vi "Test Latch when pressed.vi"(11 "Error in":errorcluster) -> (15 "Error out":errorcluster)   [LabVIEW 2020, in "Mechanical Actions Tests.lvlib"]
doc: "This VI is used to test latch when pressed function"
uses:
  Mechanical Actions Tests.lvlib
  <vilib>/addons/_JKI Toolkits/Caraya/classes/Test Suite/Define Test Suite (JUnit Report).vi
  <vilib>/SLL Drona/APIs/Stimulus/ControlValue/SetValueAuto.vi
  <vilib>/SLL Drona/APIs/Assert/AssertControlValue/Equal.vi
  <vilib>/SLL Drona/APIs/Stimulus/VI/CloseVI.vi
  <vilib>/Utility/error.llb/Error Cluster From Error Code.vi
  <vilib>/ErrorRing/Error Ring.xnode
  <vilib>/addons/_JKI Toolkits/Caraya/classes/Test Suite/Test Suite.lvclass
  <vilib>/addons/_JKI Toolkits/Caraya/classes/Test/Test.lvclass
  <vilib>/SLL Drona/Drona.lvlib
  <vilib>/SLL Drona/APIs/Stimulus/ControlValue/ControlValue.lvlib
  <vilib>/SLL Drona/APIs/Assert/AssertControlValue/AssertControlValue.lvlib
  <vilib>/Wiresmith Technology/G CLI/CLI Class/CLI.lvclass
  <vilib>/SLL Drona/APIs/Stimulus/VI/VI.lvlib
panel:
  # "LATCH WHEN PRESSED TEST"
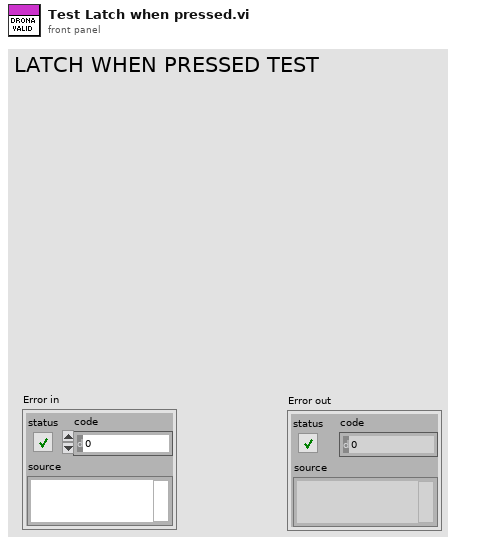
[diagram p1: front panel]
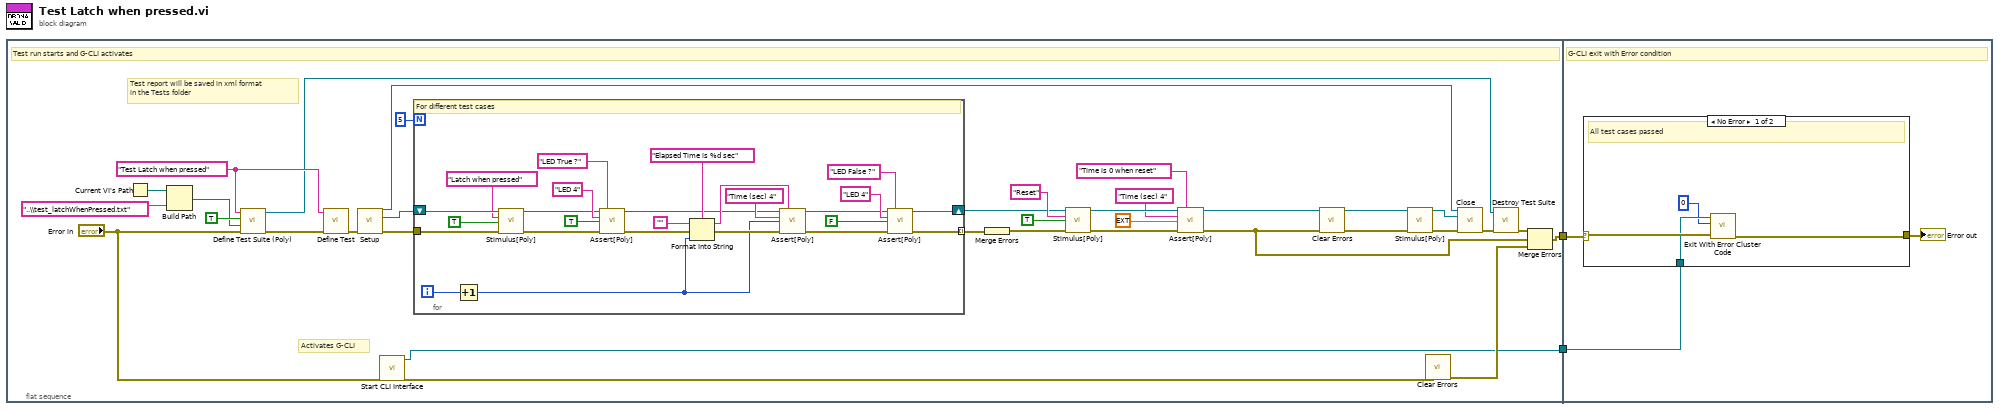
[diagram p0: block diagram]
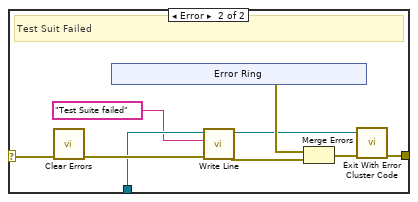
[diagram p2: hidden frame]
diagram:
  n1 = flat-sequence {
    tunnel: [w18] -> w2
    tunnel: [w5] -> w1
    tunnel: w2 -> [w64]
    tunnel: w1 -> [w62]
    frame #0 {
      w14 = "Test Latch when pressed" ("Label (VI Title)")
      # "Test report will be saved in xml format\nin the Tests folder"
      # "Activates G-CLI"
      # "Test run starts and G-CLI activates"
      n2 = Current VI's Path() -> (path=w12:path)
      n3 = Build Path(base path=w12, name or relative path="..\\test_latchWhenPressed.txt") -> (appended path=w10:path)
      n4 = call-poly <vilib>:"Define Test Suite (Poly).vi"("error in (no error)"="Error in", "Report Path"=w10, "Interactive"=TRUE, "Label (VI Title)"=w14) -> ("error out"=w16:errorcluster, "Test Suite"=w7:refnum<class "Test Suite.lvclass">)  [unwired: 5 in, 1 out]
      n5 = call <vilib>:"Define Test.vi"("error in (no error)"=w16, "Label (VI Title)"=w14) -> ("error out"=w36:errorcluster)  [unwired: 8 in, 1 out]
      n6 = call <vilib>:"Setup.vi"("error in"=w36) -> ("Application Ref"=w25:refnum<vi>, "VI Reference Out"=w35:refnum<vi>, "error out"=w23:errorcluster)  [unwired: 12 in]
      n7 = call <vilib>:"Start CLI Interface.vi"("error in (no error)"="Error in") -> ("error out"=w6:errorcluster, "CLI out"=w5:refnum<class "CLI.lvclass">)  [unwired: 7 in, 2 out]
      n8 = for {
        N: 5 -> [_]
        shift-right: [w37] -> w27
        shift-left: w35 -> [w60]
        tunnel: w23 -> [w61]
        tunnel: [w38] -> w26 mode=indexing
        i -> [w50]
        # "For different test cases"
        n9 = Increment(x=w50) -> (x+1=w46:i32)
        n10 = call-poly <vilib>:"Stimulus[Poly].vi"("VI Reference In"=w60, "Control Path"="Latch when pressed", "Value (Signaling)"=TRUE, "error in"=w61) -> ("VI Reference Out"=w43:refnum<vi>, "error out"=w44:errorcluster)  [unwired: 10 in]
        n11 = call-poly <vilib>:"Assert[Poly].vi"("VI Reference In"=w43, "Test Label"="LED True ?" ("Label"), "Control Path"="LED 4", "Control Value"=TRUE, "Error In"=w44) -> ("VI Reference Out"=w41:refnum<vi>, "Error Out"=w42:errorcluster)  [unwired: 9 in]
        n12 = Format Into String(format string="Elapsed Time is %d sec", initial string="", error in=w42, w46) -> (resulting string=w45:string, error out=w49:errorcluster)
        n13 = call-poly <vilib>:"Assert[Poly].vi"("VI Reference In"=w41, "Test Label"=w45, "Control Path"="Time (sec) 4", "Control Value"=w46, "Error In"=w49) -> ("VI Reference Out"=w40:refnum<vi>, "Error Out"=w39:errorcluster)  [unwired: 9 in]
        n14 = call-poly <vilib>:"Assert[Poly].vi"("VI Reference In"=w40, "Test Label"="LED False ?" ("Label"), "Control Path"="LED 4", "Control Value"=FALSE, "Error In"=w39) -> ("VI Reference Out"=w37:refnum<vi>, "Error Out"=w38:errorcluster)  [unwired: 9 in]
      }
      n15 = Merge Errors(w26) -> (w24:errorcluster)
      n16 = call-poly <vilib>:"Stimulus[Poly].vi"("VI Reference In"=w27, "Control Path"="Reset", "Value (Signaling)"=TRUE, "error in"=w24) -> ("VI Reference Out"=w34:refnum<vi>, "error out"=w33:errorcluster)  [unwired: 10 in]
      n17 = call-poly <vilib>:"Assert[Poly].vi"("VI Reference In"=w34, "Test Label"="Time is 0 when reset" ("Label"), "Control Path"="Time (sec) 4", "Control Value"=ext 0.0, "Error In"=w33) -> ("VI Reference Out"=w20:refnum<vi>, "Error Out"=w4:errorcluster)  [unwired: 9 in]
      n18 = call <vilib>:"Clear Errors.vi"("error in (no error)"=w4) -> ("error out"=w3:errorcluster)  [unwired: 5 in, 1 out]
      n19 = call-poly <vilib>:"Stimulus[Poly].vi"("VI Reference In"=w20, "error in"=w3) -> ("VI Reference Out"=w19:refnum<vi>, "error out"=w21:errorcluster)  [unwired: 12 in]
      n20 = call <vilib>:"Clear Errors.vi"("error in (no error)"=w6) -> ("error out"=w17:errorcluster)  [unwired: 5 in, 1 out]
      n21 = call <vilib>:"Close.vi"("Application Ref"=w25, "VI Reference"=w19, "error in"=w21) -> ("error out"=w9:errorcluster)  [unwired: 12 in]
      n22 = call-dynamic "Destroy Test Suite.vi"("error in (no error)"=w9, "Test Suite in"=w7) -> ("error out"=w8:errorcluster)  [unwired: 8 in, 1 out]
      n23 = Merge Errors(w8, w4, w17) -> (w18:errorcluster)
    }
    frame #1 {
      # "G-CLI exit with Error condition"
      n24 = case shown="No Error" w64 {
        selector: w64 -> [w68 w76]
        tunnel: [w67 w77] -> w63
        tunnel: w62 -> [w66 w74]
        frame No Error {
          # "All test cases passed"
          n25 = call <vilib>:"Exit With Error Cluster Code.vi"("error in (no error)"=w68, "No Error Code (0)"=0, "CLI in"=w66) -> ("error out"=w67:errorcluster)  [unwired: 8 in]
        }
        frame Error {
          # "Test Suit Failed"
          n26 = call <vilib>:"Clear Errors.vi"("error in (no error)"=w76) -> ("error out"=w75:errorcluster)  [unwired: 5 in, 1 out]
          n27 = xnode "Error Ring"() -> ("error out"=w72:errorcluster)
          n28 = call <vilib>:"Write Line.vi"("error in (no error)"=w75, "Text to Write"="Test Suite failed", "CLI in"=w74) -> ("error out"=w71:errorcluster, "CLI out"=w69:refnum<class "CLI.lvclass">)  [unwired: 7 in]
          n29 = Merge Errors(w72, w71) -> (w70:errorcluster)
          n30 = call <vilib>:"Exit With Error Cluster Code.vi"("error in (no error)"=w70, "CLI in"=w69) -> ("error out"=w77:errorcluster)  [unwired: 9 in]
        }
      }
      "Error out" <- w63
    }
  }
